vi "HMI Loop.vi"(7 "Expo":dbl(slide) scale=0.0..10.0, 8 "error in (no error)":errorcluster, 10 "Steering Frame in":T3, 11 "Device in":T4={"device ID"=refnum, "Device Name"="Logitech Extreme 3D", "axis info"={"X axis"=[], "Y axis"=[], "Z axis"=[], "X axis rotation"=[], "Y axis rotation"=[], "Z axis rotation"=[], "U axis"=[], "V axis"=[]}}) -> (0 "error out":errorcluster, 2 "Steering Frame out":T3, 3 "Device Out":T4={"device ID"=refnum, "Device Name"="Logitech Extreme 3D", "axis info"={"X axis"=[], "Y axis"=[], "Z axis"=[], "X axis rotation"=[], "Y axis rotation"=[], "Z axis rotation"=[], "U axis"=[], "V axis"=[]}})   [LabVIEW 2012]
uses:
  <vilib>/robotics/Steering/Class Type Definitions/Mecanum Steering Frame.ctl
  <vilib>/robotics/Steering/Mecanum Steering Frame/NI_Robotics_Mecanum Steering Frame.lvclass
  <vilib>/robotics/Steering/Class Type Definitions/Differential Steering Frame.ctl
  <vilib>/robotics/Steering/Differential Steering Frame/NI_Robotics_Differential Steering Frame.lvclass
  <vilib>/Utility/inputDevices.llb/joystickAcquire.vi
  <vilib>/robotics/Steering/Class Type Definitions/NI_Robotics_Steering Class Types.lvlib
panel:
  out "direction info":T5
  out "button info":T6
  out "axis info":T7
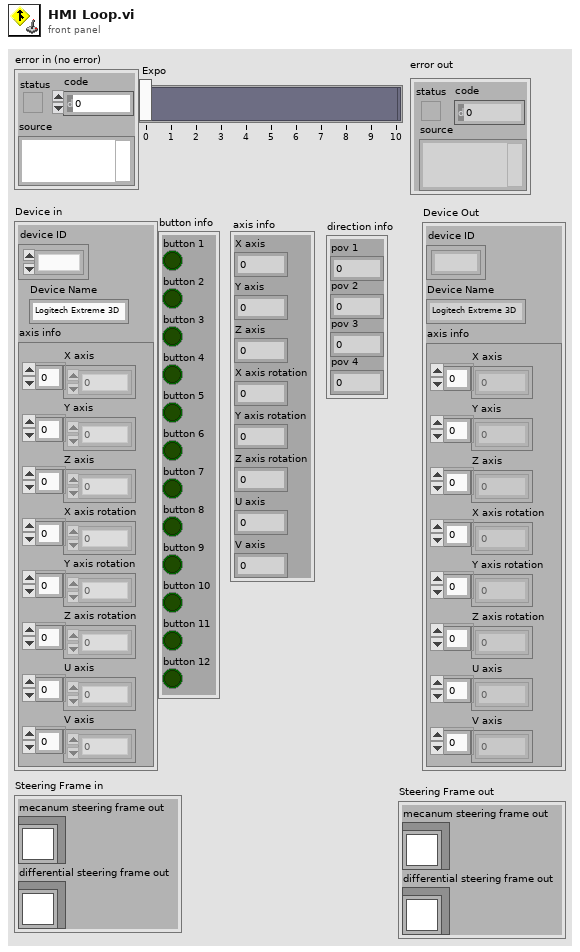
[diagram p1: front panel]
types:
  T1 = typedef "NI_Robotics_Steering Class Types.lvlib/Mecanum Steering Frame.ctl" = refnum<class "NI_Robotics_Mecanum Steering Frame.lvclass">
  T2 = typedef "NI_Robotics_Steering Class Types.lvlib/Differential Steering Frame.ctl" = refnum<class "NI_Robotics_Differential Steering Frame.lvclass">
  T3 = cluster{"mecanum steering frame out":T1, "differential steering frame out":T2}
  T4 = cluster{"device ID":refnum<k1>, "Device Name":string, "axis info":cluster{"X axis":dbl[], "Y axis":dbl[], "Z axis":dbl[], "X axis rotation":dbl[], "Y axis rotation":dbl[], "Z axis rotation":dbl[], "U axis":dbl[], "V axis":dbl[]}}
  T5 = cluster{"pov 1":i32, "pov 2":i32, "pov 3":i32, "pov 4":i32}
  T6 = cluster{"button 1":bool, "button 2":bool, "button 3":bool, "button 4":bool, "button 5":bool, "button 6":bool, "button 7":bool, "button 8":bool, "button 9":bool, "button 10":bool, "button 11":bool, "button 12":bool, "button 13":bool, "button 14":bool, "button 15":bool, "button 16":bool, "button 17":bool, "button 18":bool, "button 19":bool, "button 20":bool, "button 21":bool, "button 22":bool, "button 23":bool, "button 24":bool, "button 25":bool, "button 26":bool, "button 27":bool, "button 28":bool, "button 29":bool, "button 30":bool, "button 31":bool, "button 32":bool}
  T7 = cluster{"X axis":i32, "Y axis":i32, "Z axis":i32, "X axis rotation":i32, "Y axis rotation":i32, "Z axis rotation":i32, "U axis":i32, "V axis":i32}
  T8 = cluster{"X axis":dbl, "Y axis":dbl, "Z axis":dbl, "X axis rotation":dbl, "Y axis rotation":dbl, "Z axis rotation":dbl, "U axis":dbl, "V axis":dbl}
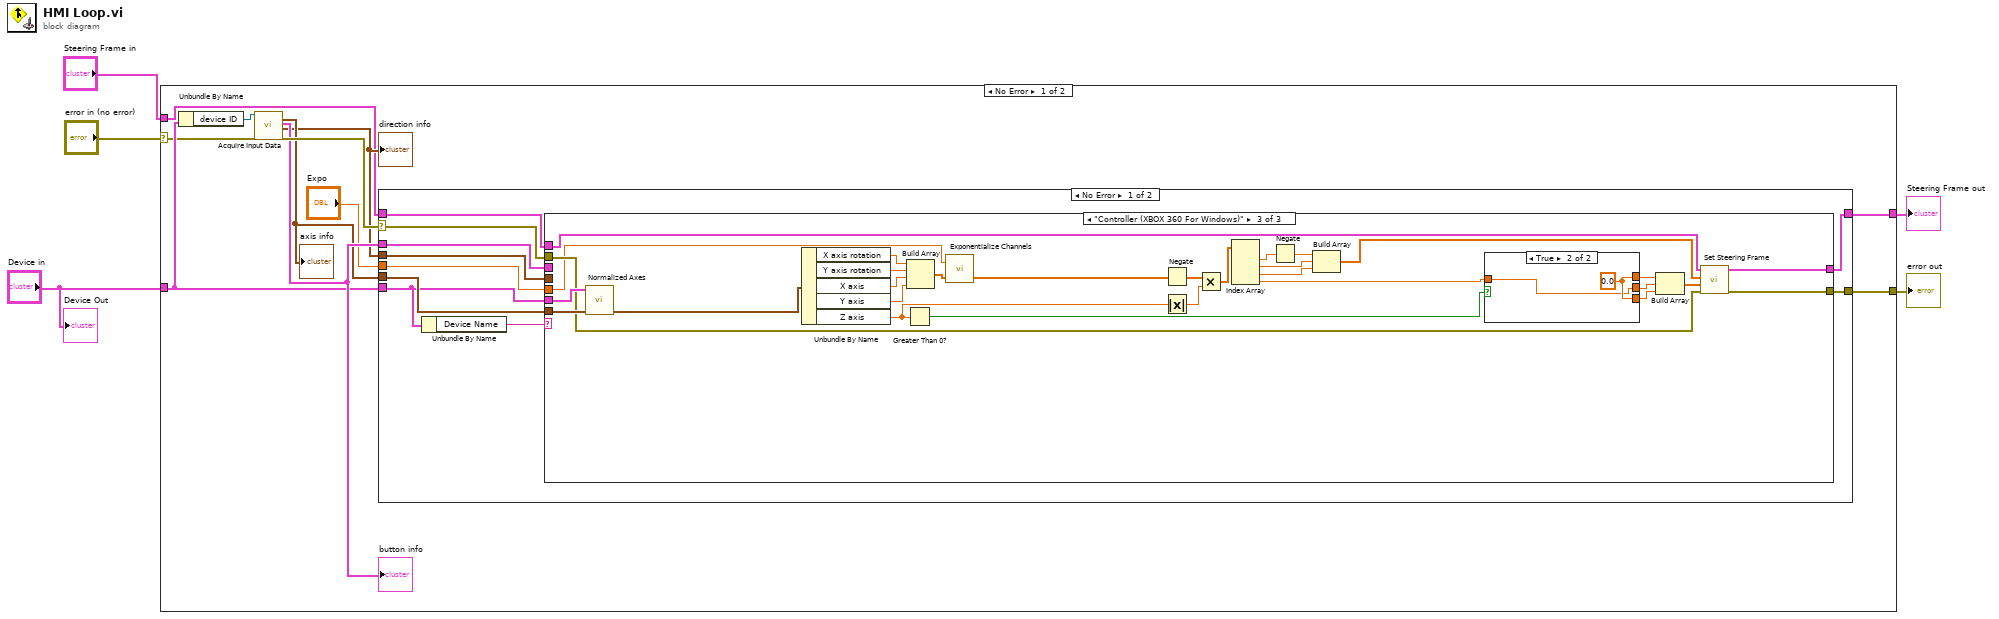
[diagram p0: block diagram]
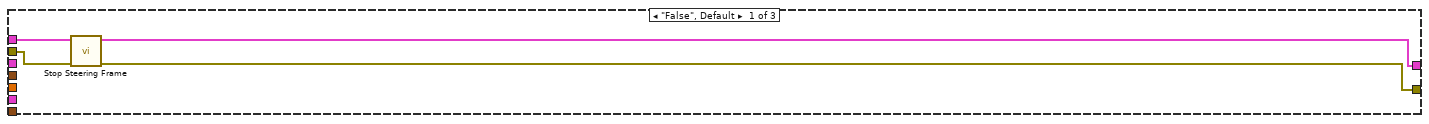
[diagram p2: hidden frame]
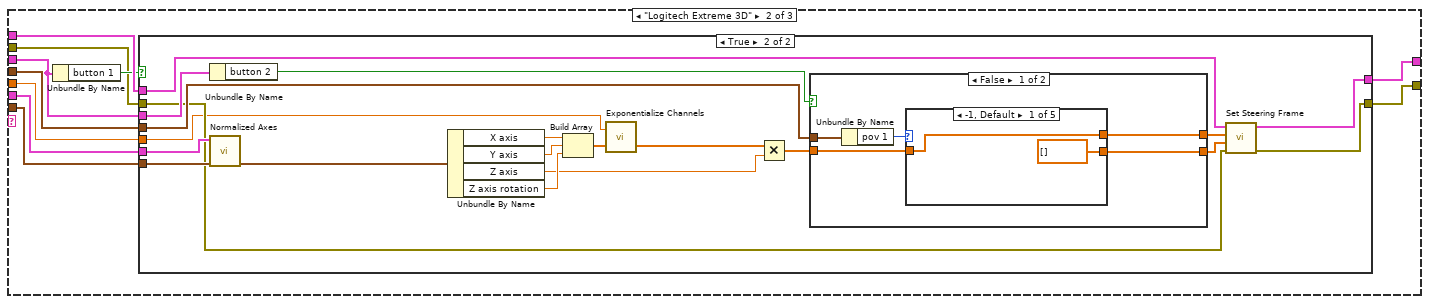
[diagram p3: hidden frame]
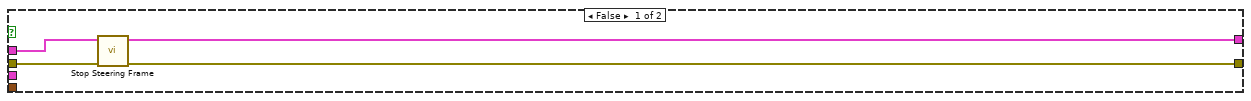
[diagram p4: hidden frame]
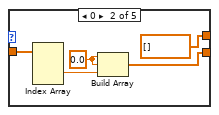
[diagram p5: hidden frame]
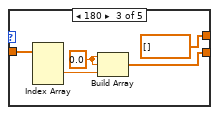
[diagram p6: hidden frame]
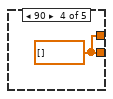
[diagram p7: hidden frame]
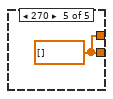
[diagram p8: hidden frame]
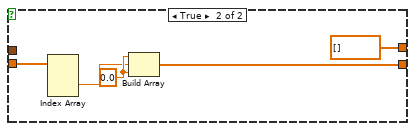
[diagram p9: hidden frame]
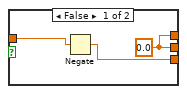
[diagram p10: hidden frame]
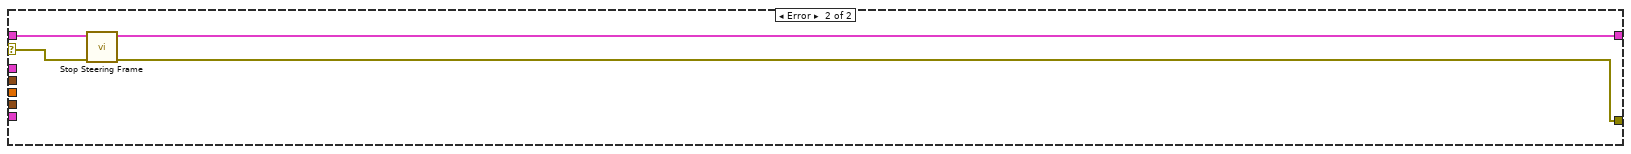
[diagram p11: hidden frame]
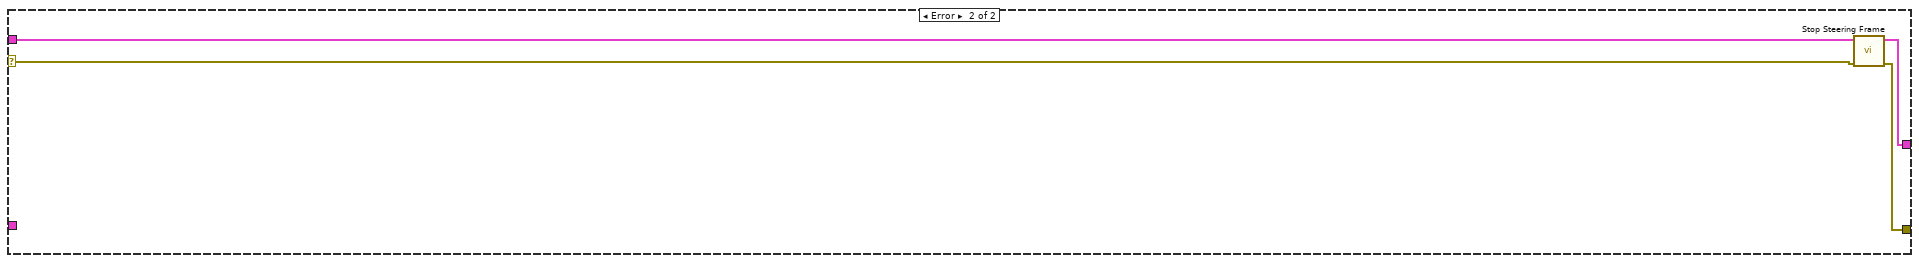
[diagram p12: hidden frame]
diagram:
  n1 = case shown="No Error" "error in (no error)" {
    selector: "error in (no error)" -> [w9 w128]
    tunnel: [w8 w130] -> w5
    tunnel: "Device in" -> [w11 _]
    tunnel: "Steering Frame in" -> [w10 w127]
    tunnel: [w7 w129] -> w1
    frame No Error {
      n2 = Unbundle By Name(w11) -> ("device ID"=w15:refnum<k1>)
      n3 = call-poly <vilib>:"Acquire Input Data.vi"("device ID"=w15, "error in (no error)"=w9) -> ("axis info"=w13:T7, "button info"=w14:T6, "direction info"=w12:T5, "error out"=w16:errorcluster)  [unwired: 13 in, 1 out]
      "axis info" <- w13
      "direction info" <- w12
      "button info" <- w14
      n4 = case shown="No Error" w16 {
        selector: w16 -> [w20 w126]
        tunnel: w14 -> [w26 _]
        tunnel: w13 -> [w25 _]
        tunnel: w12 -> [w24 _]
        tunnel: w11 -> [w22 _]
        tunnel: w10 -> [w21 w125]
        tunnel: [w19 w123] -> w8
        tunnel: [w18 w124] -> w7
        tunnel: "Expo" -> [w17 _]
        frame No Error {
          n5 = Unbundle By Name(w22) -> ("Device Name"=w23:string)
          n6 = case shown="\"Controller (XBOX 360 For Windows)\"" w23 {
            tunnel: w26 -> [_ w36 _]
            tunnel: w25 -> [_ w40 w117]
            tunnel: w24 -> [_ w38 _]
            tunnel: w22 -> [_ w39 w116]
            tunnel: w21 -> [w29 w37 w115]
            tunnel: w20 -> [w30 w34 w114]
            tunnel: [w27 w33 w113] -> w19
            tunnel: [w28 w32 w112] -> w18
            tunnel: w17 -> [_ w31 w89]
            frame "False", Default {
              n7 = call "Stop Steering Frame.vi"("error in (no error)"=w30, "Steering Frame in"=w29) -> ("error out"=w27:errorcluster, "Steering Frame out"=w28:T3)  [unwired: 8 in]
            }
            frame "Logitech Extreme 3D" {
              n8 = Unbundle By Name(w36) -> ("button 1"=w35:bool)
              n9 = case shown="True" w35 {
                tunnel: w40 -> [_ w60]
                tunnel: w39 -> [_ w52]
                tunnel: w38 -> [_ w56]
                tunnel: w36 -> [_ w58]
                tunnel: w37 -> [w41 w48]
                tunnel: [w42 w49] -> w32
                tunnel: w34 -> [w44 w51]
                tunnel: [w43 w50] -> w33
                tunnel: w31 -> [_ w45]
                frame False {
                  n10 = call "Stop Steering Frame.vi"("error in (no error)"=w44, "Steering Frame in"=w41) -> ("error out"=w43:errorcluster, "Steering Frame out"=w42:T3)  [unwired: 8 in]
                }
                frame True {
                  n11 = Unbundle By Name(w58) -> ("button 2"=w57:bool)
                  n12 = call "Normalized Axes.vi"("axis in"=w60, "Device in"=w52) -> ("axis out"=w62:T8)  [unwired: 8 in, 1 out]
                  n13 = Unbundle By Name(w62) -> ("X axis"=w63:dbl, "Y axis"=w64:dbl, "Z axis"=w55:dbl, "Z axis rotation"=w59:dbl)
                  n14 = Build Array(w63, w64, w59) -> (w61:dbl[])
                  n15 = call "Exponentialize Channels.vi"("Channels in"=w61, "Expo"=w45) -> ("Channels out"=w54:dbl[])  [unwired: 1 in]
                  n16 = Multiply(x=w54, y=w55) -> (x*y=w53:dbl[])
                  n17 = case shown="False" w57 {
                    tunnel: [w69 dbl[] []] -> w47
                    tunnel: [w68 w85] -> w46
                    tunnel: w56 -> [w67 _]
                    tunnel: w53 -> [w65 w87]
                    frame False {
                      n18 = Unbundle By Name(w67) -> ("pov 1"=w66:i32)
                      n19 = case shown="-1, Default" w66 {
                        tunnel: w65 -> [w71 w76 w81 _ _]
                        tunnel: [w71 dbl[] [] dbl[] [] w82 w83] -> w69
                        tunnel: [dbl[] [] w72 w77 w82 w83] -> w68
                        frame -1, Default {
                        }
                        frame 0 {
                          w74 = 0.0 ("element")
                          n20 = Index Array(array=w76) -> (element #2=w75:dbl)  [unwired: 3 in, 2 out]
                          n21 = Build Array(w74, w74, w75) -> (w72:dbl[])
                        }
                        frame 180 {
                          w79 = 0.0 ("element")
                          n22 = Index Array(array=w81) -> (element #2=w80:dbl)  [unwired: 3 in, 2 out]
                          n23 = Build Array(w79, w79, w80) -> (w77:dbl[])
                        }
                        frame 90 {
                          w82 = dbl[] []
                        }
                        frame 270 {
                          w83 = dbl[] []
                        }
                      }
                    }
                    frame True {
                      w86 = 0.0 ("element")
                      n24 = Index Array(array=w87) -> (element #2=w84:dbl)  [unwired: 3 in, 2 out]
                      n25 = Build Array(w86, w84, w86) -> (w85:dbl[])
                    }
                  }
                  n26 = call "Set Steering Frame.vi"("error in (no error)"=w51, "differential frame velocity"=w46, "mecanum frame velocity"=w47, "Steering Frame in"=w48) -> ("error out"=w50:errorcluster, "Steering Frame out"=w49:T3)  [unwired: 6 in]
                }
              }
            }
            frame "Controller (XBOX 360 For Windows)" {
              n27 = call "Normalized Axes.vi"("axis in"=w117, "Device in"=w116) -> ("axis out"=w111:T8)  [unwired: 8 in, 1 out]
              n28 = Unbundle By Name(w111) -> ("X axis rotation"=w107:dbl, "Y axis rotation"=w106:dbl, "X axis"=w105:dbl, "Y axis"=w104:dbl, "Z axis"=w99:dbl)
              n29 = Greater Than 0?(x=w99) -> (x > 0?=w98:bool)
              n30 = Build Array(w107, w106, w105, w104) -> (w103:dbl[])
              n31 = call "Exponentialize Channels.vi"("Channels in"=w103, "Expo"=w89) -> ("Channels out"=w110:dbl[])  [unwired: 1 in]
              n32 = Negate(x=w110) -> (-x=w93:dbl[])
              n33 = Absolute Value(x=w99) -> (abs(x)=w100:dbl)
              n34 = Multiply(x=w93, y=w100) -> (x*y=w109:dbl[])
              n35 = Index Array(array=w109) -> (element #1=w102:dbl, element #2=w91:dbl, element #3=w92:dbl, element #4=w97:dbl)  [unwired: 4 in]
              n36 = Negate(x=w102) -> (-x=w90:dbl)
              n37 = Build Array(w90, w91, w92) -> (w101:dbl[])
              n38 = case shown="True" w98 {
                tunnel: w97 -> [w120 w121]
                tunnel: [w119 w122] -> w96
                tunnel: [w119 w121] -> w95
                tunnel: [w118 w122] -> w94
                frame False {
                  w119 = 0.0 ("element")
                  n39 = Negate(x=w120) -> (-x=w118:dbl)
                }
                frame True {
                  w122 = 0.0 ("element")
                }
              }
              n40 = Build Array(w96, w95, w94) -> (w108:dbl[])
              n41 = call "Set Steering Frame.vi"("error in (no error)"=w114, "differential frame velocity"=w108, "mecanum frame velocity"=w101, "Steering Frame in"=w115) -> ("error out"=w113:errorcluster, "Steering Frame out"=w112:T3)  [unwired: 6 in]
            }
          }
        }
        frame Error {
          n42 = call "Stop Steering Frame.vi"("error in (no error)"=w126, "Steering Frame in"=w125) -> ("error out"=w123:errorcluster, "Steering Frame out"=w124:T3)  [unwired: 8 in]
        }
      }
    }
    frame Error {
      n43 = call "Stop Steering Frame.vi"("error in (no error)"=w128, "Steering Frame in"=w127) -> ("error out"=w130:errorcluster, "Steering Frame out"=w129:T3)  [unwired: 8 in]
    }
  }
  "error out" <- w5
  "Steering Frame out" <- w1
  "Device Out" <- "Device in"
